vi "Prober_ValidCoordinate.vi"(8 "error in (no error)":errorcluster, 9 "Axis":enum16{"X", "Y", "Z", "Theta"}(ring), 10 "Coordinate IN":i32, 11 "TeslaVeloxProbeStation in":refnum<class "TeslaVeloxProbeStation.lvclass">) -> (0 "error out":errorcluster, 2 "Is Valid?":bool, 3 "TeslaVeloxProbeStation out":refnum<class "TeslaVeloxProbeStation.lvclass">)   [LabVIEW 2018, in "TeslaVeloxProbeStation.lvclass"]
uses:
  TeslaVeloxProbeStation.lvclass
  TeslaVeloxProbeStation.lvclass/TeslaVeloxProbeStation.ctl
panel:
  out "Coordinate system":enum16{"Cartesian", "X as index"}(ring)
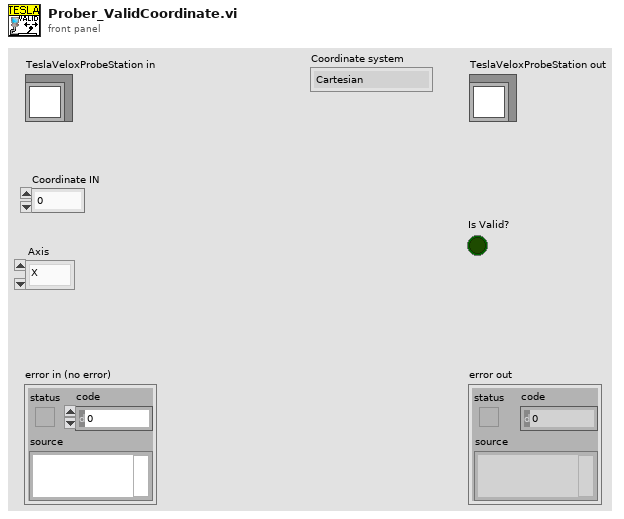
[diagram p1: front panel]
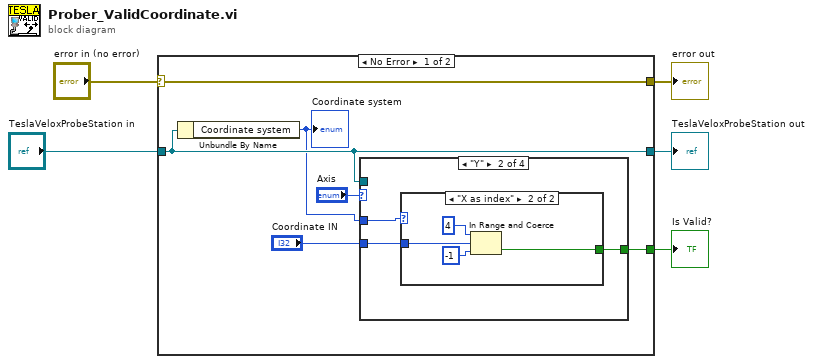
[diagram p0: block diagram]
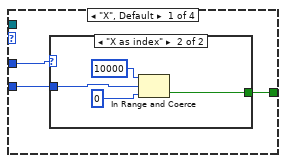
[diagram p2: hidden frame]
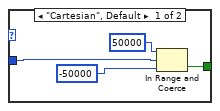
[diagram p3: hidden frame]
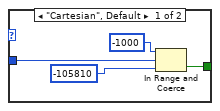
[diagram p4: hidden frame]
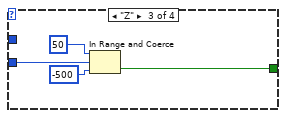
[diagram p5: hidden frame]
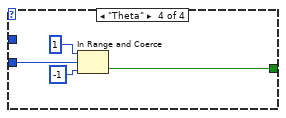
[diagram p6: hidden frame]
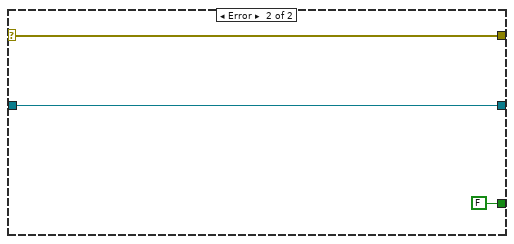
[diagram p7: hidden frame]
diagram:
  n1 = case shown="No Error" "error in (no error)" {
    selector: "error in (no error)" -> [w6 w42]
    tunnel: [w11 FALSE] -> w3
    tunnel: [w6 w42] -> w1
    tunnel: "TeslaVeloxProbeStation in" -> [w8 w43]
    tunnel: [w8 w43] -> w2
    frame No Error {
      n2 = Unbundle By Name(w8) -> ("Coordinate system"=w7:enum16{"Cartesian", "X as index"})
      "Coordinate system" <- w7
      n3 = case shown="\"Y\"" "Axis" {
        tunnel: "Coordinate IN" -> [w14 w25 w35 w39]
        tunnel: [w13 w24 w34 w38] -> w11
        tunnel: w8 -> [_ _ _ _]
        tunnel: w7 -> [w12 w23 _ _]
        frame "X", Default {
          n4 = case shown="\"X as index\"" w12 {
            tunnel: w14 -> [w17 w22]
            tunnel: [w15 w19] -> w13
            frame "Cartesian", Default {
              n5 = In Range and Coerce(upper limit=50000, x=w17, lower limit=-50000) -> (In Range?=w15:bool)  [unwired: 1 out]
            }
            frame "X as index" {
              n6 = In Range and Coerce(upper limit=10000, x=w22, lower limit=0) -> (In Range?=w19:bool)  [unwired: 1 out]
            }
          }
        }
        frame "Y" {
          n7 = case shown="\"X as index\"" w23 {
            tunnel: w25 -> [w27 w32]
            tunnel: [w26 w30] -> w24
            frame "Cartesian", Default {
              n8 = In Range and Coerce(upper limit=-1000, x=w27, lower limit=-105810) -> (In Range?=w26:bool)  [unwired: 1 out]
            }
            frame "X as index" {
              n9 = In Range and Coerce(upper limit=4, x=w32, lower limit=-1) -> (In Range?=w30:bool)  [unwired: 1 out]
            }
          }
        }
        frame "Z" {
          n10 = In Range and Coerce(upper limit=50, x=w35, lower limit=-500) -> (In Range?=w34:bool)  [unwired: 1 out]
        }
        frame "Theta" {
          n11 = In Range and Coerce(upper limit=1, x=w39, lower limit=-1) -> (In Range?=w38:bool)  [unwired: 1 out]
        }
      }
    }
    frame Error {
    }
  }
  "error out" <- w1
  "TeslaVeloxProbeStation out" <- w2
  "Is Valid?" <- w3
